vi "get_settings_cluster.vi"(8 "error in (no error)":errorcluster, 11 "GenericPlugin in":refnum<class "TrajectoryDL110413StraightLine.lvclass">) -> (0 "error out":errorcluster, 2 "settings cluster":variant, 3 "GenericPlugin out":refnum<class "TrajectoryDL110413StraightLine.lvclass">)   [LabVIEW 2010, in "TrajectoryDL110413StraightLine.lvclass"]
uses:
  TrajectoryDL110413StraightLine.lvclass
  TrajectoryDL110413StraightLine.lvclass/TrajectoryDL110413StraightLine.ctl
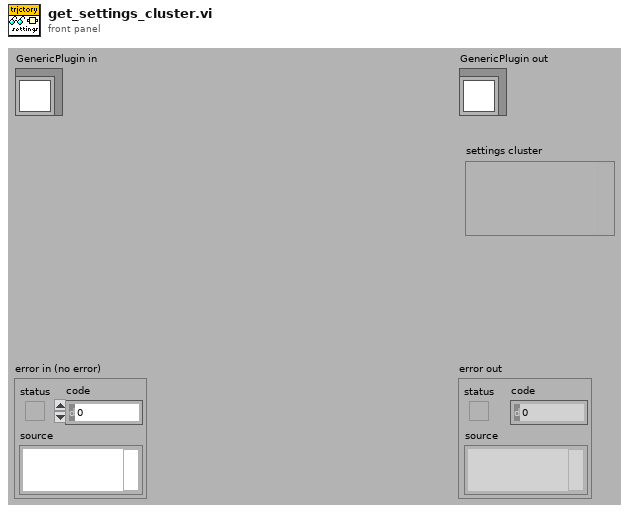
[diagram p1: front panel]
types:
  T1 = typedef "TrajectoryDL110413StraightLine.lvclass/settings_cluster.ctl" = cluster{"number of pixels":dbl}
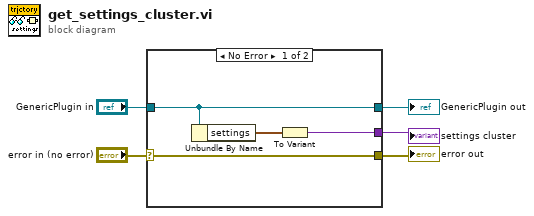
[diagram p0: block diagram]
diagram:
  n1 = case shown="No Error" "error in (no error)" {
    selector: "error in (no error)" -> [w9 w11]
    tunnel: [w9 w11] -> w4
    tunnel: "GenericPlugin in" -> [w6 w10]
    tunnel: [w7 _] -> w2
    tunnel: [w6 w10] -> w1
    frame No Error {
      n2 = Unbundle By Name(w6) -> ("settings"=w8:T1)
      n3 = To Variant(anything=w8) -> (Variant=w7:variant)
    }
    frame Error {
    }
  }
  "error out" <- w4
  "GenericPlugin out" <- w1
  "settings cluster" <- w2
